vi "Auto Match.vi"() -> ()   [LabVIEW 2017]
panel:
  out "Number of iterations":i32
  out "Current number":u32
  in  "Number to match":u32=50 max=1000 step=1
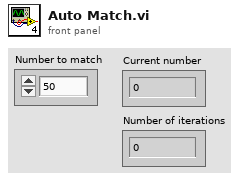
[diagram p1: front panel]
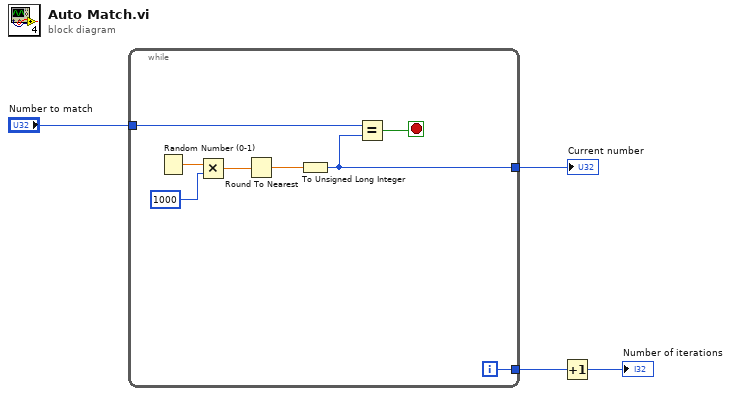
[diagram p0: block diagram]
diagram:
  n1 = while {
    tunnel: [w5] -> w4
    tunnel: [w7] -> w1
    tunnel: "Number to match" -> [w6]
    i -> [w7]
    stop <- w8 stop-if-true
    n2 = Random Number (0-1)() -> (number: 0 to 1=w12:dbl)
    n3 = Multiply(x=w12, y=1000) -> (x*y=w10:dbl)
    n4 = Round To Nearest(number=w10) -> (nearest integer value=w9:dbl)
    n5 = To Unsigned Long Integer(number=w9) -> (unsigned 32bit integer=w5:u32)
    n6 = Equal?(x=w6, y=w5) -> (x = y?=w8:bool)
  }
  "Current number" <- w4
  n7 = Increment(x=w1) -> (x+1=→"Number of iterations":i32)
